vi "Dequeue Message.vi"(0 "Message Queue":refnum<queue> caption="메시지 큐", 5 "타임아웃(ms) (-1)":i32, 11 "error in (no error)":errorcluster caption="에러 입력(에러 없음)") -> (4 "dup Message Queue":refnum<queue> caption="메시지 큐 복제", 6 "Message":string caption="메시지", 8 "Message Data":variant caption="메시지 데이터", 10 "타임아웃?":bool, 15 "error out":errorcluster caption="에러 출력")   [LabVIEW 2018, in "Message Queue.lvlib"]
doc: "이 VI는 메시지를 메시지 큐에서 제거합니다."
uses:
  Message Queue.lvlib
  Message Cluster.ctl
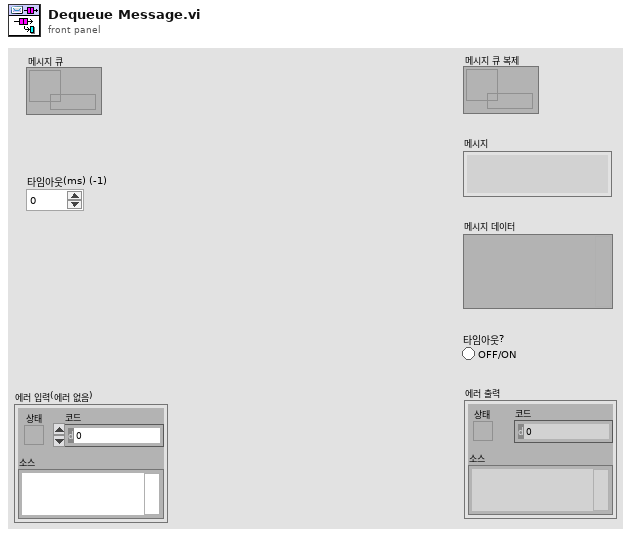
[diagram p1: front panel]
types:
  T1 = typedef "Message Queue.lvlib/Message Cluster.ctl" = cluster{"Message":string, "Message Data":variant}
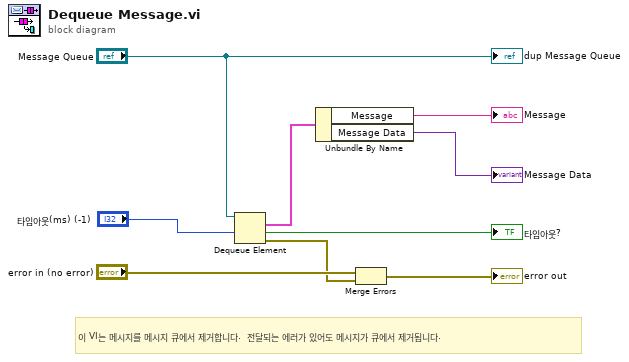
[diagram p0: block diagram]
diagram:
  # "이 VI는 메시지를 메시지 큐에서 제거합니다.  전달되는 에러가 있어도 메시지가 큐에서 제거됩니다."
  n1 = Dequeue Element(queue="Message Queue", timeout in ms (-1)="타임아웃(ms) (-1)") -> (element=w6:T1, timed out?=→"타임아웃?":bool, error out=w3:errorcluster)  [unwired: 1 in, 1 out]
  n2 = Unbundle By Name(w6) -> ("Message"=→"Message":string, "Message Data"=→"Message Data":variant)
  n3 = Merge Errors("error in (no error)", w3) -> (→"error out":errorcluster)
  "dup Message Queue" <- "Message Queue"
